vi "Read.vi"(8 "error in (no error)":errorcluster, 11 "object in":refnum<class "Pressure-Transducer.lvclass">) -> (0 "error out":errorcluster, 2 "Data":dbl[](array[numeric]), 3 "object out":refnum<class "Pressure-Transducer.lvclass">)   [LabVIEW 2021, in "Pressure-Transducer.lvclass"]
doc: "Read converted data from modbus Reg"
uses:
  Pressure-Transducer.lvclass
  Modbus-Instr_class/Modbus-Instr.lvclass
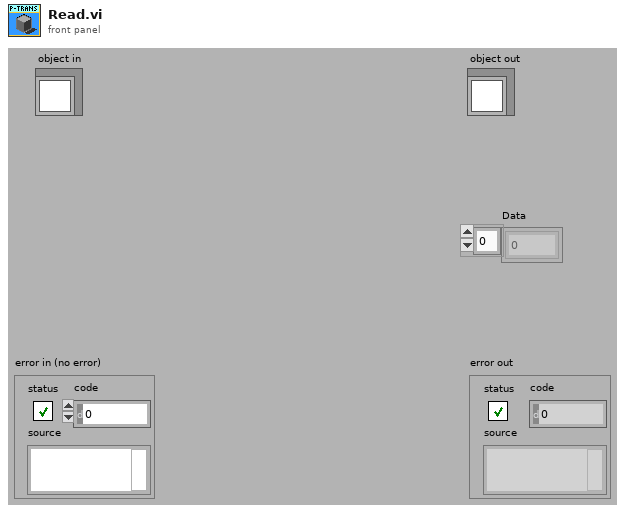
[diagram p1: front panel]
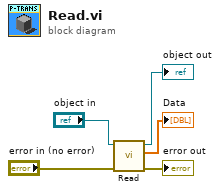
[diagram p0: block diagram]
diagram:
  n1 = call-parent "Read.vi"("error in (no error)"="error in (no error)", "object in"="object in") -> ("error out"=→"error out":errorcluster, "Data"=→"Data":dbl[], "object out"=→"object out":refnum<class "Pressure-Transducer.lvclass">)  [unwired: 7 in]
